vi "XY Plot Matrix.vi"() -> ()   [LabVIEW 2017, in "2D_Merge.lvlib"]
uses:
  <vilib>/Math Plots/2D Math Plots/Merge VIs/2D_Merge.lvlib
  <vilib>/Math Plots/2D Math Plots/XY Plot Matrix/XY Plot Matrix XCtrl/XY Plot Matrix.xctl
  <vilib>/Math Plots/2D Math Plots/XY Plot Matrix/XY Plot Matrix Datatype/XY Plot Matrix Datatype.lvclass
panel:
  out "XY Plot Matrix":refnum<class "XY Plot Matrix Datatype.lvclass">[](xcontrol)
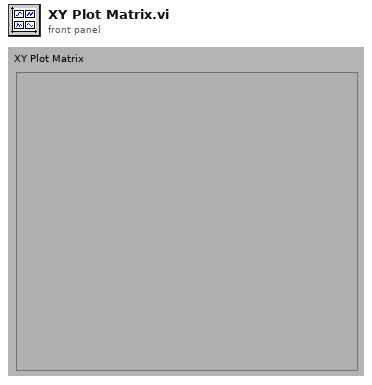
[diagram p1: front panel]
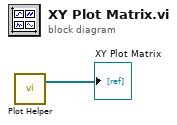
[diagram p0: block diagram]
diagram:
  n1 = call <vilib>:"Plot Helper.vi"() -> ("2D Plotmatrix Class Obj Array out"=→"XY Plot Matrix":refnum<class "XY Plot Matrix Datatype.lvclass">[])  [unwired: 4 in, 7 out]
